vi "SetHeader.vi"(8 "error in (no error)":errorcluster, 10 "Header in":refnum<class "Collection.lvclass">, 11 "Table in":refnum<class "Table.lvclass">) -> (0 "error out":errorcluster, 3 "Table out":refnum<class "Table.lvclass">)   [LabVIEW 2021, in "LvMarkdown.lvlib" / "Table.lvclass"]
uses:
  Table.lvclass
  Table.lvclass/Table.ctl
  Collection/Collection.lvclass
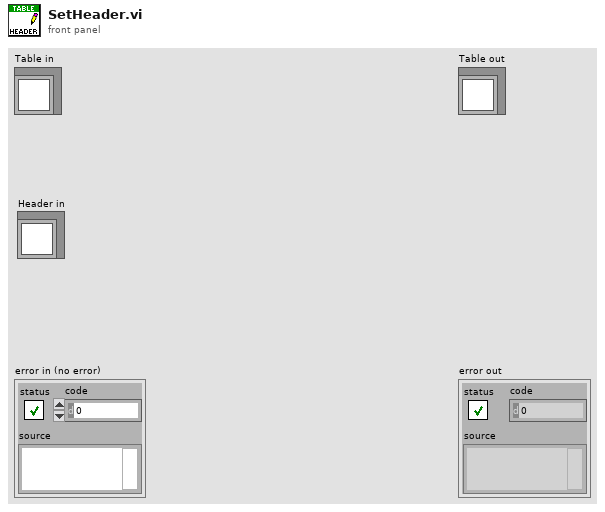
[diagram p1: front panel]
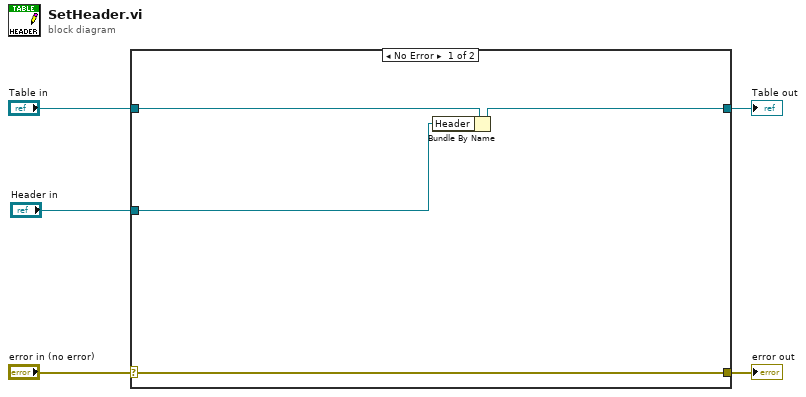
[diagram p0: block diagram]
diagram:
  n1 = case shown="No Error" "error in (no error)" {
    selector: "error in (no error)" -> [w8 w11]
    tunnel: [w8 w11] -> w4
    tunnel: [w7 w10] -> w2
    tunnel: "Table in" -> [w9 w10]
    tunnel: "Header in" -> [w6 _]
    frame No Error {
      n2 = Bundle By Name(cluster=w9, "Header"=w6) -> (w7:refnum<class "Table.lvclass">)
    }
    frame Error {
    }
  }
  "error out" <- w4
  "Table out" <- w2
